vi "CNT Get Counter.vi"(8 "error in (no error)":errorcluster, 9 "Channel":u8, 10 "DevIndex":i32, 11 "DevType":i32) -> (0 "error out":errorcluster, 2 "function return":i32, 3 "pCounterValue":u32)   [LabVIEW 2012, in "ControlCNT.lvlib"]
doc: "int WINAPI CNT_GetCounter(int DevType, int DevIndex, unsigned char Channel, unsigned int *pCounterValue);"
uses:
  ControlCNT.lvlib
  Ginkgo_Driver.dll
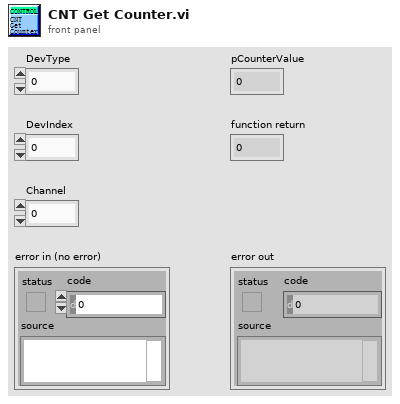
[diagram p1: front panel]
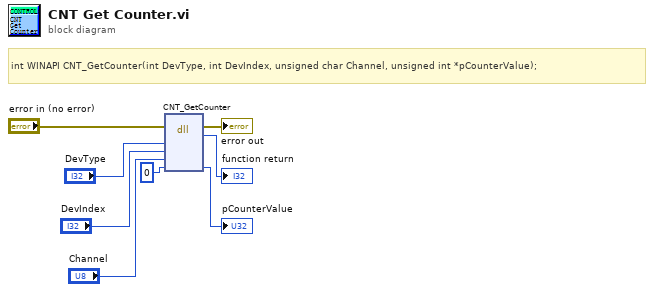
[diagram p0: block diagram]
diagram:
  # "int WINAPI CNT_GetCounter(int DevType, int DevIndex, unsigned char Channel, unsigned int *pCounterValue);"
  n1 = dll-call lib="E:/Project/vt_ginkgo/truck/Ginkgo Driver/vs2010/Ginkgo_USB-I2C_API_v2.0.3.0/lib/labview_64bit/ControlCNT/Ginkgo_Driver.*" fn="CNT_GetCounter"(error in="error in (no error)", "DevType"="DevType", "DevIndex"="DevIndex", "Channel"="Channel", "pCounterValue"=u32 0) -> (error out=→"error out":errorcluster, →"function return":i32, "pCounterValue"=→"pCounterValue":u32)  [unwired: 5 in, 1 out]
